vi "读取CH1.vi"(8 "error in":errorcluster, 11 "Resource Name":refnum<k15>="DAQ::1") -> (0 "error out":errorcluster, 3 "Waveform From Scope":waveform(dbl)[](graph) caption="Waveform from Scope")   [LabVIEW 2018]
uses:
  <instrlib>/niScope/Configure/Trigger/niScope Configure Trigger Edge.vi
  <instrlib>/niScope/Acquire/niScope Multi Read WDT.vi
panel:
  in  "Channel(s)":string="0" caption="Channel"
  in  "Vertical Range (V)":dbl=5.0 format="%_3g"
  in  "Min. Sample Rate":dbl=10000000.0 min=10.0 max=60000000.0 format="%#_6p"
  in  "Min Record Length":i32=40000
  in  "Vertical Coupling":i32(ring)=1 items=["AC", "DC", "Ground"]
  in  "Trigger Slope":i32(ring) items=["Positive", "Negative"]
  in  "Coupling":u16(ring)=1 items=["AC"=0, "DC"=1, "HF Reject"=3, "LF Reject"=4, "AC Plus HF Reject"=1001]
  in  "Trigger Level (V)":dbl=0.5 caption="Trigger Level" format="%.2f"
  in  "Trigger Modifier":i32(ring)=2 items=["None"=1, "Auto Trigger"=2]
  in  "Input Impedance":u32(ring) items=["1 mega ohm"=0, "50 ohms"=2]
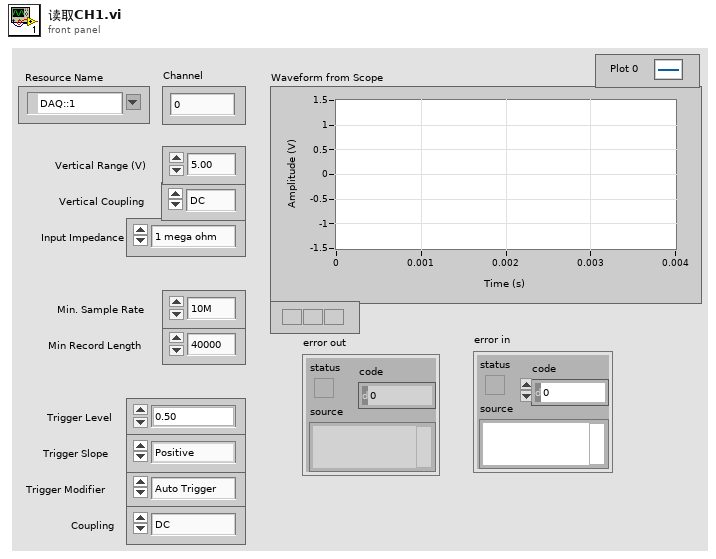
[diagram p1: front panel]
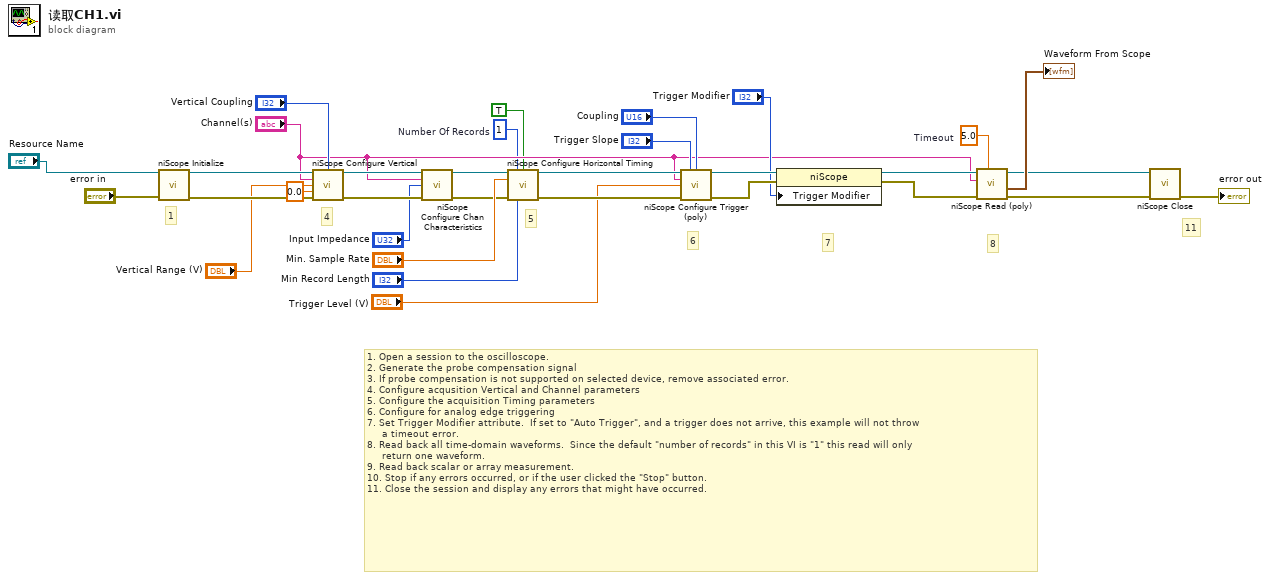
[diagram p0: block diagram]
diagram:
  w7 = 1  # Number Of Records
  w14 = 5.0  # Timeout
  # "8"
  # "6"
  # "5"
  # "4"
  # "7"
  # "11"
  # "1"
  # "1. Open a session to the oscilloscope.\n2. Generate the probe compensation signal \n3. If probe compensation is not supported on selected device, remove associated error.\n4. Configure acqusition Vertical and Channel parameters\n5. Configure the acquisition Timing parameters\n6. Configure for analog edge triggering\n7. Set Trigger Modifier attribute.  If set to \"Auto Trigger\", and a trigger does not arrive, this example will not throw\n     a timeout error.\n8. Read back all time-domain waveforms.  Since the default \"number of records\" in this VI is \"1\" this read will only\n     return one waveform.\n9. Read back scalar or array measurement.\n10. Stop if any errors occurred, or if the user clicked the \"Stop\" button.\n11. Close the session and display any errors that might have occurred."
  n1 = call <instrlib>:"niScope Initialize.vi"("resource name"="Resource Name", "error in"="error in") -> ("instrument handle"=w31:refnum<k15>, "error out"=w30:errorcluster)  [unwired: 12 in]
  n2 = call <instrlib>:"niScope Configure Vertical.vi"("instrument handle"=w31, "vertical coupling"="Vertical Coupling", "channels"="Channel(s)", "vertical range"="Vertical Range (V)", "vertical offset"=0.0, "error in"=w30) -> ("instrument handle out"=w12:refnum<k15>, "error out"=w13:errorcluster)  [unwired: 8 in]
  n3 = call <instrlib>:"niScope Configure Chan Characteristics.vi"("instrument handle"=w12, "channels"="Channel(s)", "input impedance"="Input Impedance", "error in"=w13) -> ("instrument handle out"=w10:refnum<k15>, "error out"=w9:errorcluster)  [unwired: 10 in]
  n4 = call <instrlib>:"niScope Configure Horizontal Timing.vi"("instrument handle"=w10, "number of records"=w7, "enforce realtime"=TRUE ("Enforce Realtime"), "min sample rate"="Min. Sample Rate", "error in"=w9, "min record length"="Min Record Length") -> ("instrument handle out"=w24:refnum<k15>, "error out"=w25:errorcluster)  [unwired: 8 in]
  n5 = call-poly <instrlib>:"niScope Configure Trigger (poly).vi"("instrument handle"=w24, "trigger slope"="Trigger Slope", "trigger coupling"="Coupling", "trigger source"="Channel(s)", "trigger level"="Trigger Level (V)", "error in"=w25) -> ("instrument handle out"=w19:refnum<k15>, "error out"=w18:errorcluster)  [unwired: 8 in]
  n6 = property class="niScope"(reference=w19, error in=w18, "Trigger Modifier"="Trigger Modifier") -> (reference out=w15:refnum<k15>, error out=w16:errorcluster)
  n7 = call-poly <instrlib>:"niScope Read (poly).vi"("timeout"=w14, "error in"=w16, "channels"="Channel(s)", "instrument handle"=w15) -> ("error out"=w4:errorcluster, "wfm"=→"Waveform From Scope":waveform(dbl)[], "instrument handle out"=w5:refnum<k15>)  [unwired: 4 in, 1 out]
  n8 = call <instrlib>:"niScope Close.vi"("instrument handle"=w5, "error in"=w4) -> ("error out"=→"error out":errorcluster)  [unwired: 13 in]
